vi "GET_volume_by_id.vi"(4 "volume":i32, 6 "volume type":T1=enum."One Shot" caption="Enum", 8 "error in (no error)":errorcluster, 10 "volume id":i32, 11 "REST Client in":refnum<class "REST Client.lvclass">) -> (0 "error out":errorcluster, 2 "local volume":T2={"id"=0, "name"="", "sortable_name"="", "aliases"=[], "description"="", "site_detail_url"="", "count_of_issues"=0, "start_year"=0, "publisher_id"=0, "issue_ids"=[], "date_last_updated"=timestamp(0 s since 1904-01-01), "volume"=0, "cv_id"="", "volume type"=enum."One Shot"}, 3 "REST Client out":refnum<class "REST Client.lvclass">)   [LabVIEW 2024, in "CV_RESTful_Lib.lvlib"]
uses:
  CV_RESTful_Lib.lvlib
  <vilib>/addons/_JKI.lib/REST Client/classes/REST Client/REST Client.lvclass
  typedefs/local_volume--cluster.ctl
  CV_Shared_Library/volume.type--enum.ctl
  <vilib>/addons/_JKI.lib/REST Client/classes/REST Client/HTTP Header.ctl
  <vilib>/NI/Advanced HTTP Client/Header--Combo Box.ctl
  typedefs/cv_volume--cluster.ctl
  typedefs/cv_volume.results--cluster.ctl
  typedefs/cv_volume.issue--cluster.ctl
  typedefs/cv_volume.publisher--cluster.ctl
  <vilib>/NI/Advanced HTTP Client/Session.lvclass
  <userlib>/_OpenG.lib/string/string.llb/openg_string.lvlib
  <vilib>/addons/_JKI.lib/Serialization/JSON/JKI JSON Serialization.lvlib
  CV_Shared_Library/CV_Shared_Library.lvlib
panel:
  out "Status String":string
  out "Status Code":u16
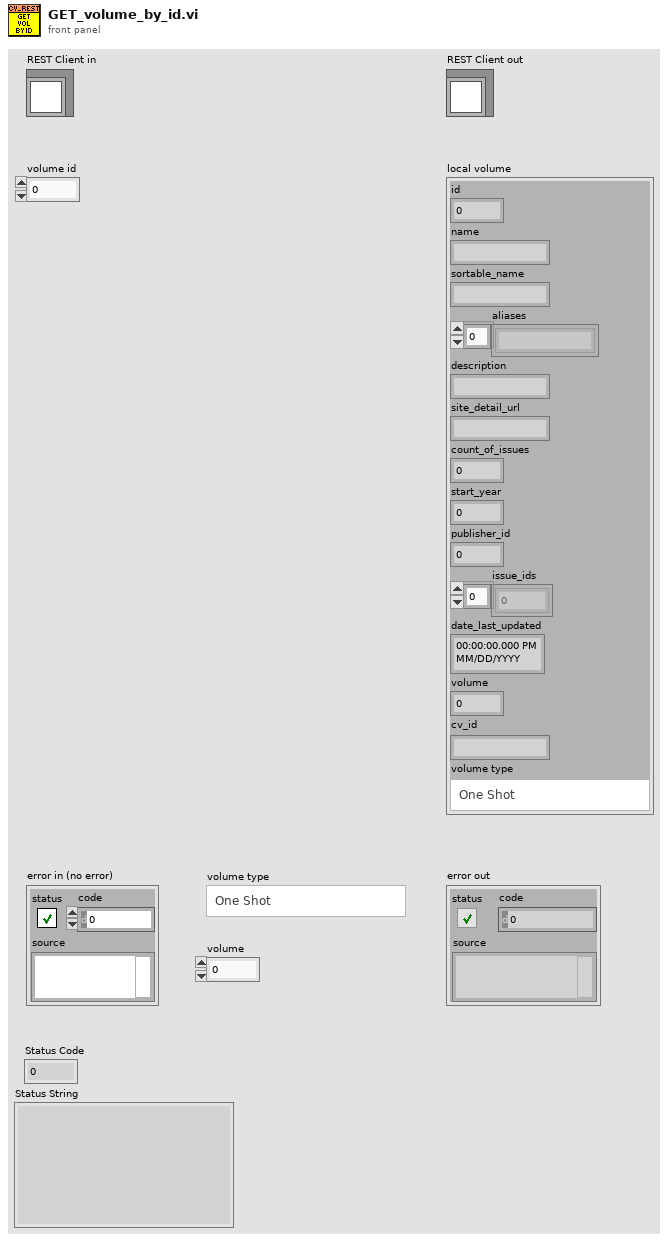
[diagram p1: front panel]
types:
  T1 = typedef "CV_Shared_Library.lvlib/volume.type--enum.ctl" = enum16{"Ongoing", "Limited Series", "Annual", "One Shot", "Reprint/Document", "Star Comics", "Epic Comics"}
  T2 = typedef "CV_RESTful_Lib.lvlib/local_volume--cluster.ctl" = cluster{"id":i32, "name":string, "sortable_name":string, "aliases":string[], "description":string, "site_detail_url":string, "count_of_issues":i32, "start_year":i32, "publisher_id":i32, "issue_ids":i32[], "date_last_updated":timestamp, "volume":i32, "cv_id":string, "volume type":T1}
  T3 = typedef "CV_RESTful_Lib.lvlib/cv_volume--cluster.ctl" = cluster{"error":string, "limit":i32, "offset":i32, "number_of_page_results":i32, "number_of_total_results":i32, "status_code":i32, "results":T4}
  T4 = typedef "CV_RESTful_Lib.lvlib/cv_volume.results--cluster.ctl" = cluster{"aliases":string, "count_of_issues":i32, "date_last_updated":timestamp, "deck":string, "id":i32, "issues":T5[], "name":string, "publisher":T6, "site_detail_url":string, "start_year":string, "description":string}
  T5 = typedef "CV_RESTful_Lib.lvlib/cv_volume.issue--cluster.ctl" = cluster{"id":i32}
  T6 = typedef "CV_RESTful_Lib.lvlib/cv_volume.publisher--cluster.ctl" = cluster{"id":i32}
  T7 = typedef "REST Client.lvlib/REST Client.lvclass/HTTP Header.ctl" = cluster{"header":T8, "value":string}
  T8 = typedef "lib_NI_Advanced HTTP Client.lvlib/Session.lvclass/Header--Combo Box.ctl" = string
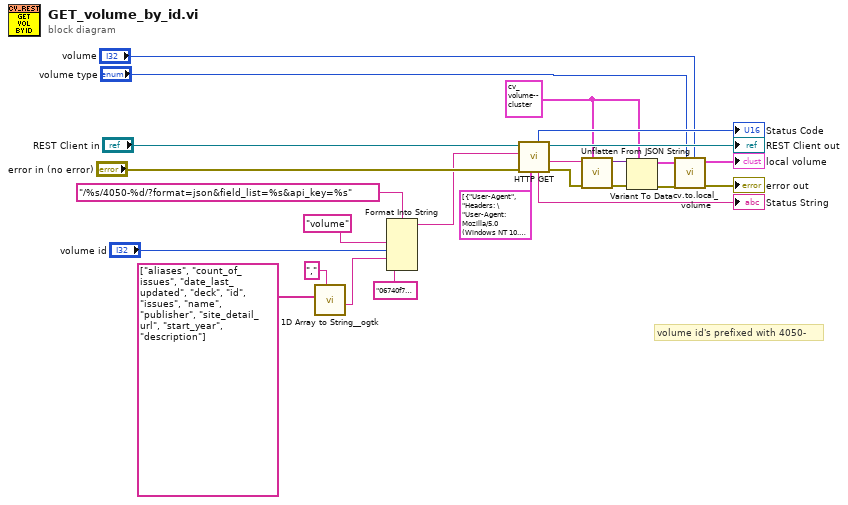
[diagram p0: block diagram]
diagram:
  w5 = T3 {"error"="", "limit"=0, "offset"=0, "number_of_page_results"=0, "number_of_total_results"=0, "status_code"=0, "results"={"aliases"="", "count_of_issues"=0, "date_last_updated"=timestamp(0 s since 1904-01-01), "deck"="", "id"=0, "issues"=[], "name"="", "publisher"={"id"=0}, "site_detail_url"="", "start_year"="", "description"=""}} ("volume")
  # "volume id's prefixed with 4050-"
  n1 = call <userlib>:"1D Array to String__ogtk.vi"("delimiter (Tab)"=",", "Array of Strings"=string[] ["aliases", "count_of_issues", "date_last_updated", "deck", "id", "issues", "name", "publisher", "site_detail_url", "start_year", "description"]) -> ("delimited string"=w16:string)  [unwired: 9 in]
  n2 = Format Into String(format string="/%s/4050-%d/?format=json&field_list=%s&api_key=%s", "volume" ("resource"), "volume id", w16, "06740f73403e0b211d597c50ea94c7f16ea5e8ea") -> (resulting string=w21:string)  [unwired: 2 in, 1 out]
  n3 = call-dynamic "HTTP GET.vi"("request specific headers"=T7[] [{"header"="User-Agent", "value"="Headers: \"User-Agent: Mozilla/5.0 (Windows NT 10.0; Win64; x64) AppleWebKit/537.36 (KHTML, like Gecko) Chrome/91.0.4472.101 Safari/537.36\""}], "error in (no error)"="error in (no error)", "Path"=w21, "REST Client in"="REST Client in") -> ("error out"=w9:errorcluster, "Response body"=w8:string, "REST Client out"=→"REST Client out":refnum<class "REST Client.lvclass">, "Status String"=→"Status String":string, "Status Code"=→"Status Code":u16)  [unwired: 2 in, 1 out]
  n4 = call <vilib>:"Unflatten From JSON String.vi"("Type and Defaults"=w5, "error in"=w9, "JSON String"=w8) -> ("error out"=w7:errorcluster, "Variant"=w6:variant)  [unwired: 7 in]
  n5 = Variant To Data(error in=w7, type=w5, Variant=w6) -> (data=w4:T3, error out=w3:errorcluster)
  n6 = call "cv.to.local_volume.vi"("volume"="volume", "volume type"="volume type", "error in (no error)"=w3, "cv volume"=w4) -> ("error out"=→"error out":errorcluster, "local volume"=→"local volume":T2)  [unwired: 6 in]
